vi "Write_NetworkStream_OCU_Override.vi"(0 "VKey":T1, 1 "NetworkStreamWriter in":refnum<class "NetworkStreamWriter.lvclass">, 5 "Mainsail Position":T4, 7 "Jib Position":T3, 9 "Rudder Setpoint":T2 min=-0.95 max=0.95 scale=1.0..-1.0, 11 "error in (no error)":errorcluster, 12 "OverrideMode":T5) -> (3 "NetworkStreamWriter out":refnum<class "NetworkStreamWriter.lvclass">, 4 "Main Position":T4, 6 "Jib Position":T3, 8 "Rudder Position":T2 min=-0.95 max=0.95 scale=1.0..-1.0, 15 "error out":errorcluster)   [LabVIEW 2013]
doc: "Takes in the key value pressed and changes the value of the main sail, jib, and rudder accordingly with the following mapping of the arrow keys (ish):\n\n\"Page Up\" -- rudder right | \"Up\" -- Main out | \"Page Down\" -- Jib out\n\"Left\" -- rudder left | \"Down\" -- Main in | \"Right\" -- Jib in\n\nIt then bundles the main sail, jib sail, and rudder override commands and sends them to the boat using NetworkStreams. It also bundles with them the override mode so the Forebrain Sense can determine which actuator setting so implement and which to ignore. Deals with coersions, becaues humans can be silly.\n\n\n\nWritten by Victoria Coleman 04/12/14"
uses:
  cRIO_Code/Data/TypeDefs/Sail Set Suggestions.ctl
  cRIO_Code/Data/TypeDefs/OverrideMode.ctl
  cRIO_Code/Data/TypeDefs/MainsailPositionIndicator.ctl
  cRIO_Code/Data/TypeDefs/JibPositionIndicator.ctl
  cRIO_Code/Data/TypeDefs/Rudder Set Suggestions.ctl
  <vilib>/event_ctls.llb/eventvkey.ctl
  Writer/NetworkStreamWriter.lvclass
  cRIO_Code/Data/TypeDefs/OverrideInformation.ctl
  OCU/CommandMessages.ctl
panel:
  in  "Sail Suggesstions":T6 {"MainSailSuggestion" min=0.0 max=1.0; "JibSailSuggestion" min=0.0 max=1.0}
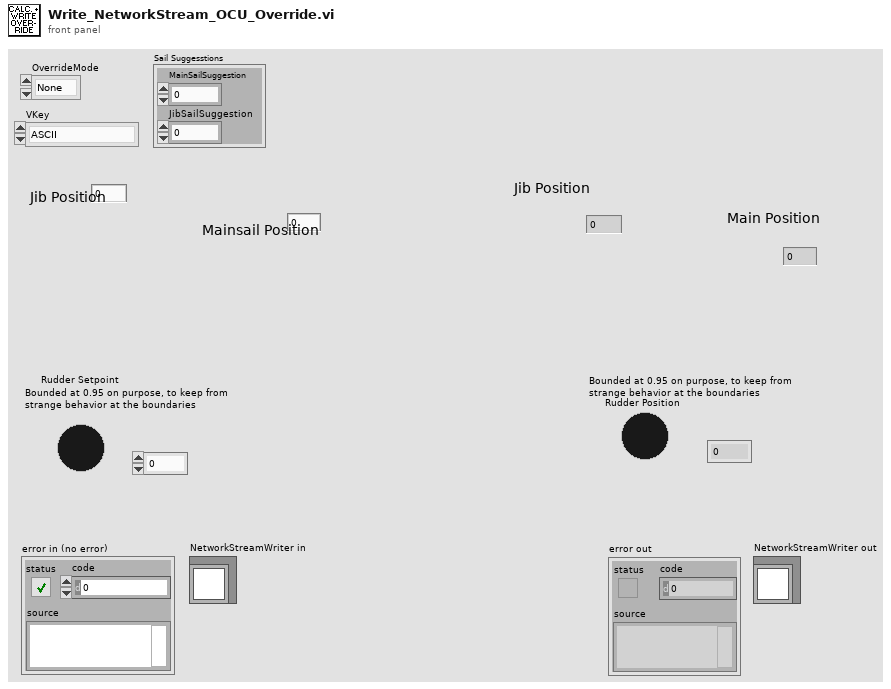
[diagram p1: front panel]
types:
  T1 = typedef "eventvkey.ctl" = enum16{"ASCII", "Enter", "Return", "Shift", "Ctrl", "Alt", "Cmd", "Opt", "Caps", "NumLock", "Clear", "Break", "Up", "Down", "Left", "Right", "Insert", "Delete", "Home", "End", "PageUp", "PageDown", "Escape", "Help", "Pause", "ScrollLock", "F1", "F2", "F3", "F4", "F5", "F6", "F7", "F8", "F9", "F10", "F11", "F12", "F13", "F14", "F15", "F16", "F17", "F18", "F19", "F20", "F21", "F22", "F23", "F24", "Play", "VolumeUp", "VolumeDown", "Mute", "Two Byte Char"}
  T2 = typedef "Rudder Set Suggestions.ctl" = dbl
  T3 = typedef "JibPositionIndicator.ctl" = dbl
  T4 = typedef "MainsailPositionIndicator.ctl" = dbl
  T5 = typedef "OverrideMode.ctl" = enum16{"None", "Rudder", "Sails", "Both"}
  T6 = typedef "Sail Set Suggestions.ctl" = cluster{"MainSailSuggestion":dbl, "JibSailSuggestion":dbl}
  T7 = typedef "CommandMessages.ctl" = enum16{"Pass", "OverrideMode", "Add mission", "Delete mission", "Change constants"}
  T8 = typedef "OverrideInformation.ctl" = cluster{"OverrideMode":T5, "SailSetting":T6, "Rudder Setpoint":T2}
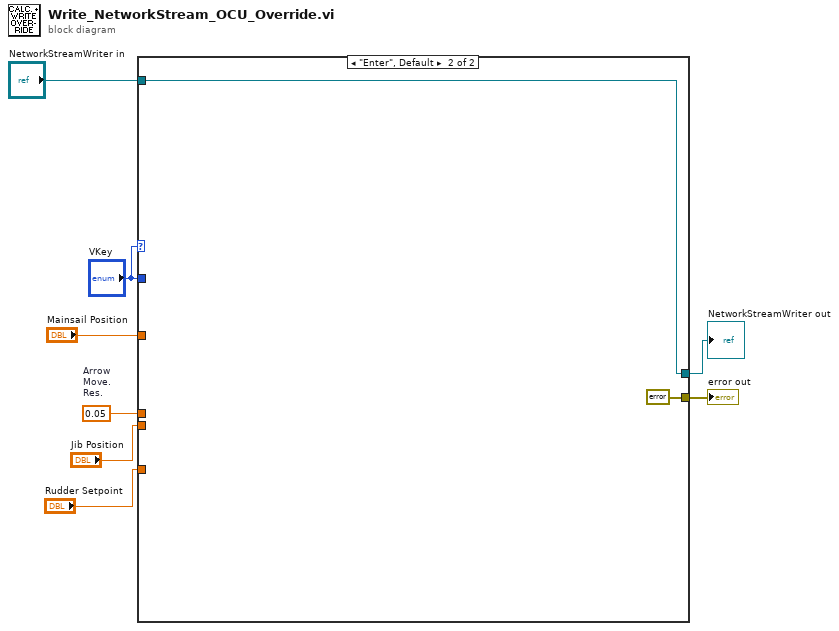
[diagram p0: block diagram]
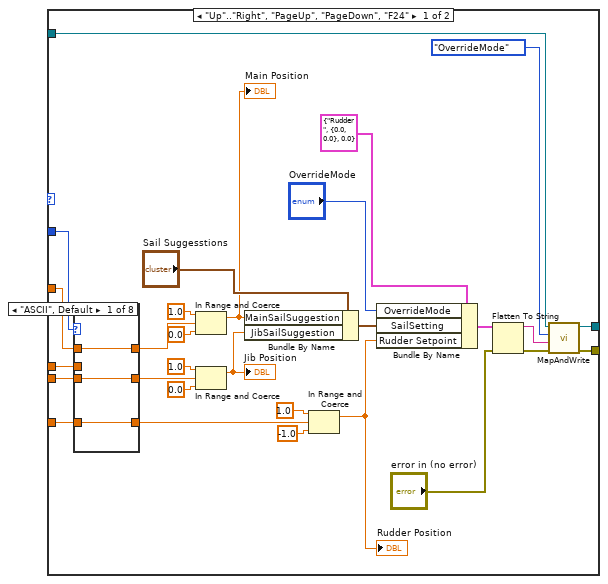
[diagram p2: hidden frame]
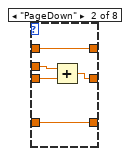
[diagram p3: hidden frame]
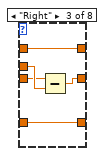
[diagram p4: hidden frame]
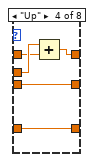
[diagram p5: hidden frame]
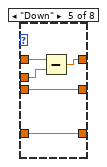
[diagram p6: hidden frame]
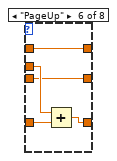
[diagram p7: hidden frame]
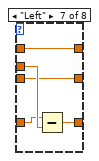
[diagram p8: hidden frame]
diagram:
  w8 = T4 0.05  # Arrow Move. Res.
  n1 = case shown="\"Enter\", Default" "VKey" {
    tunnel: w8 -> [w32 _]
    tunnel: "Jib Position" -> [w16 _]
    tunnel: "Rudder Setpoint" -> [w15 _]
    tunnel: [w13 errorcluster {"status"=FALSE, "code"=0, "source"=""} ("error out")] -> w5
    tunnel: [w12 w74] -> w4
    tunnel: "Mainsail Position" -> [w11 _]
    tunnel: "VKey" -> [w10 _]
    tunnel: "NetworkStreamWriter in" -> [w9 w74]
    frame "Up".."Right", "PageUp", "PageDown", "F24" {
      n2 = case shown="\"ASCII\", Default" w10 {
        tunnel: w15 -> [w38 w42 w48 w53 w57 w64 w69 w71]
        tunnel: w16 -> [w39 w44 w47 w51 w58 w63 w68 w72]
        tunnel: w11 -> [w40 w43 w46 w54 w60 w62 w67 w73]
        tunnel: w32 -> [_ w45 w50 w55 w59 w65 w70 _]
        tunnel: [w39 w41 w49 w51 w58 w63 w68 w72] -> w36
        tunnel: [w40 w43 w46 w52 w56 w62 w67 w73] -> w30
        tunnel: [w38 w42 w48 w53 w57 w61 w66 w71] -> w20
        frame "ASCII", Default {
        }
        frame "PageDown" {
          n3 = Add(x=w45, y=w44) -> (x+y=w41:T4)
        }
        frame "Right" {
          n4 = Subtract(x=w47, y=w50) -> (x-y=w49:T3)
        }
        frame "Up" {
          n5 = Add(x=w55, y=w54) -> (x+y=w52:T4)
        }
        frame "Down" {
          n6 = Subtract(x=w60, y=w59) -> (x-y=w56:T4)
        }
        frame "PageUp" {
          n7 = Add(x=w65, y=w64) -> (x+y=w61:T4)
        }
        frame "Left" {
          n8 = Subtract(x=w69, y=w70) -> (x-y=w66:T2)
        }
        frame "F24" {
        }
      }
      n9 = In Range and Coerce(upper limit=T4 1.0, x=w30, lower limit=T4 0.0) -> (coerced(x)=w22:T4)  [unwired: 1 out]
      "Main Position" <- w22
      n10 = In Range and Coerce(upper limit=T3 1.0, x=w36, lower limit=T3 0.0) -> (coerced(x)=w23:T3)  [unwired: 1 out]
      "Jib Position" <- w23
      n11 = Bundle By Name(cluster="Sail Suggesstions", "MainSailSuggestion"=w22, "JibSailSuggestion"=w23) -> (w28:T6)
      n12 = In Range and Coerce(upper limit=T2 1.0, x=w20, lower limit=T2 -1.0) -> (coerced(x)=w19:T2)  [unwired: 1 out]
      "Rudder Position" <- w19
      n13 = Bundle By Name(cluster=T8 {"OverrideMode"=enum."Rudder", "SailSetting"={"MainSailSuggestion"=0.0, "JibSailSuggestion"=0.0}, "Rudder Setpoint"=0.0} ("OverrideInfo"), "OverrideMode"="OverrideMode", "SailSetting"=w28, "Rudder Setpoint"=w19) -> (w27:T8)
      n14 = Flatten To String(anything=w27, error in (no error)="error in (no error)") -> (data string=w25:string, error out=w26:errorcluster)  [unwired: 2 in, 1 out]
      n15 = call "MapAndWrite.vi"("error in (no error)"=w26, "String_Cast_of_Info"=w25, "Commands"=CommandMessages."OverrideMode", "NetworkStreamWriter in"=w9) -> ("error out"=w13:errorcluster, "NetworkStreamWriter out"=w12:refnum<class "NetworkStreamWriter.lvclass">)  [unwired: 2 in]
    }
    frame "Enter", Default {
    }
  }
  "error out" <- w5
  "NetworkStreamWriter out" <- w4
